vi "ResetECU.vi"(7 "CAN Log Path":path, 8 "错误输入（无错误）":errorcluster, 10 "Boolean":bool, 11 "CAN ID":T1={"RequestID"=0, "ResponseID"=1946, "FunctionID"=2015} {"FunctionID" format="%.0x"; "ResponseID" format="%.0x"; "RequestID" format="%.0x"}) -> (0 "错误输出":errorcluster, 3 "Pass？":bool)   [LabVIEW 2024]
uses:
  Controls/CAN ID.ctl
panel:
  out "Data":u8[](array[numeric]) format="%.0x"
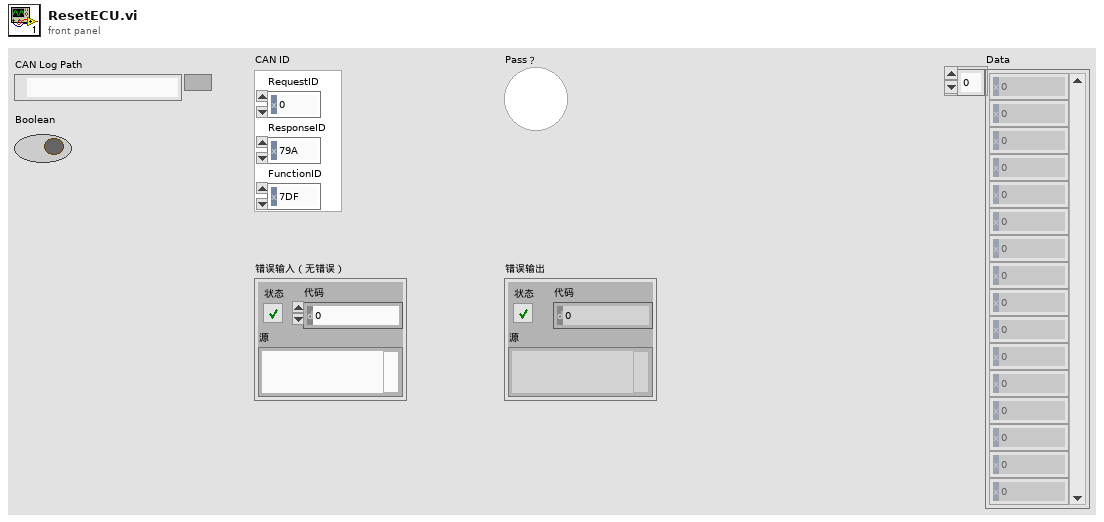
[diagram p1: front panel]
types:
  T1 = typedef "CAN ID.ctl" = cluster{"RequestID":i32, "ResponseID":i32, "FunctionID":i32}
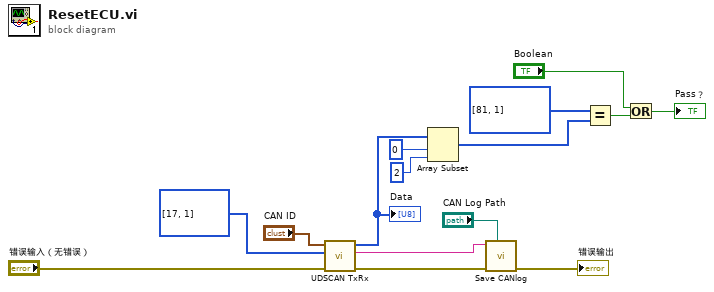
[diagram p0: block diagram]
diagram:
  n1 = call "UDSCAN TxRx.vi"("error in (no error)"="错误输入（无错误）", "Data In"=u8[] [17, 1], "CAN ID"="CAN ID") -> ("error out"=w6:errorcluster, "CAN Text"=w9:string, "Data Out"=w8:u8[])  [unwired: 6 in]
  "Data" <- w8
  n2 = Array Subset(array=w8, index=0, length=2) -> (w11:u8[])
  n3 = call "Save CANlog.vi"("CAN Log Path"="CAN Log Path", "错误输入"=w6, "text"=w9) -> ("错误输出"=→"错误输出":errorcluster)  [unwired: 8 in]
  n4 = Equal?(x=u8[] [81, 1] ("Data In"), y=w11) -> (x = y?=w3:bool)
  n5 = Or(x="Boolean", y=w3) -> (x .or. y?=→"Pass？":bool)
